vi "Configure Math Function Average.vi"(8 "error in (no error)":errorcluster, 9 "Number of Averages (8: 8)":i32(ring)=8 items=["2"=2, "4"=4, "8"=8, "16"=16, "32"=32, "64"=64, "128"=128, "256"=256, "512"=512, "1024"=1024, "2048"=2048, "4096"=4096, "8192"=8192, "16384"=16384, "32768"=32768, "65536"=65536], 10 "Math Function Index (1: Math Function 1)":i32(ring)=1 items=["Math Function 1"=1, "Math Function 2"=2, "Math Function 3"=3, "Math Function 4"=4], 11 "VISA resource name":refnum<visa-resource-name>) -> (0 "error out":errorcluster, 3 "VISA resource name out":refnum<visa-resource-name>)   [LabVIEW 2010, in "Agilent 2000 3000 X-Series.lvlib"]
doc: "Thins VI sets the number of waveforms to be averaged together."
uses:
  <instrlib>/Agilent 2000 3000 X-Series/Agilent 2000 3000 X-Series.lvlib
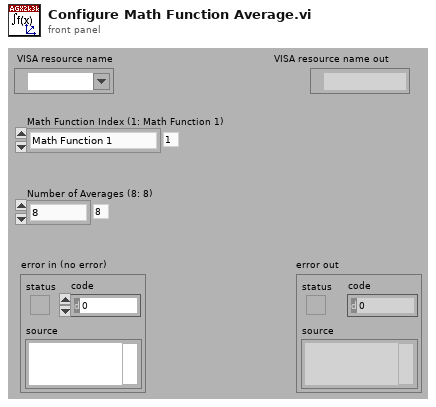
[diagram p1: front panel]
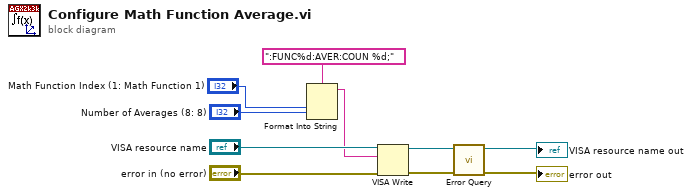
[diagram p0: block diagram]
diagram:
  n1 = Format Into String(format string=":FUNC%d:AVER:COUN %d;", "Math Function Index (1: Math Function 1)", "Number of Averages (8: 8)") -> (resulting string=w3:string)  [unwired: 2 in, 1 out]
  n2 = VISA Write(VISA resource name="VISA resource name", write buffer=w3, error in (no error)="error in (no error)") -> (VISA resource name out=w9:refnum<visa-resource-name>, error out=w8:errorcluster)  [unwired: 1 out]
  n3 = call <instrlib>:"Error Query.vi"("error in (no error)"=w8, "VISA resource name"=w9) -> ("error out"=→"error out":errorcluster, "VISA resource name out"=→"VISA resource name out":refnum<visa-resource-name>)  [unwired: 8 out]
